vi "Camera_close.vi"(8 "error in":errorcluster) -> (0 "error out":errorcluster, 1 "关闭设备返回值":i32)   [LabVIEW 2016]
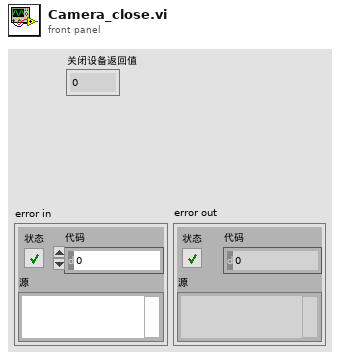
[diagram p1: front panel]
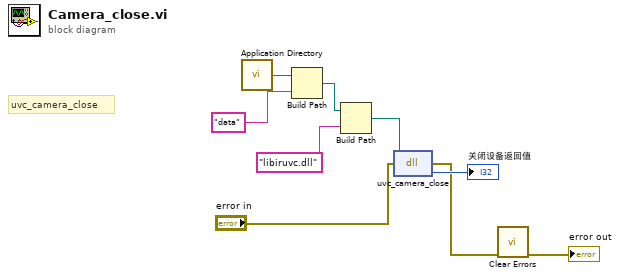
[diagram p0: block diagram]
diagram:
  # "uvc_camera_close"
  n1 = call <vilib>:"Application Directory.vi"() -> ("Application Directory"=w8:path)
  n2 = Build Path(base path=w8, name or relative path="data") -> (appended path=w6:path)
  n3 = Build Path(base path=w6, name or relative path="libiruvc.dll") -> (appended path=w9:path)
  n4 = dll-call lib="D:/libiruvc_0.3.3/windows/x64/dll/libiruvc.dll" fn="uvc_camera_close"(path in=w9, error in="error in") -> (error out=w2:errorcluster, "return type"=→"关闭设备返回值":i32)  [unwired: 1 in, 1 out]
  n5 = call <vilib>:"Clear Errors.vi"("error in (no error)"=w2) -> ("error out"=→"error out":errorcluster)  [unwired: 5 in, 1 out]
